vi "Initialize.vi"(8 "error in (no error)":errorcluster, 11 "VISA resource name":refnum<visa-resource-name>) -> (0 "error out":errorcluster, 3 "VISA resource name out":refnum<visa-resource-name>)   [LabVIEW 2023, in "JY-SPEX-TRIAX.lvlib"]
doc: "Establishes communication with the spectrometer; if the spectrometer hasn't yet been initialized, it does so. Generally, you need to call the Initialize VI only if the spectrometer has been powered off."
uses:
  JY-SPEX-TRIAX.lvlib
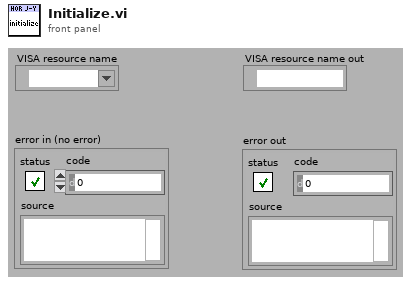
[diagram p1: front panel]
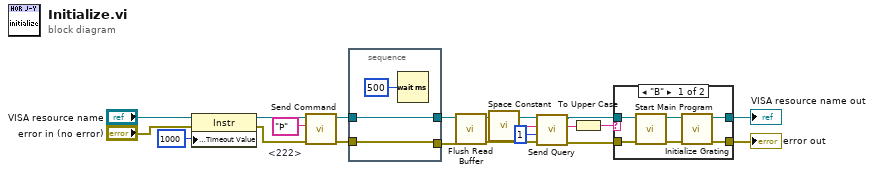
[diagram p0: block diagram]
diagram:
  w9 = "Þ"  # <222>
  n1 = property class="Instr"(reference="VISA resource name", error in="error in (no error)", "General Settings:Timeout Value"=u32 1000) -> (reference out=w14:refnum<visa-resource-name>, error out=w12:errorcluster)
  n2 = call "Send Command.vi"("error in (no error)"=w12, "write buffer"=w9, "VISA resource name"=w14) -> ("error out"=w11:errorcluster, "VISA resource name out"=w13:refnum<visa-resource-name>)  [unwired: 7 out]
  n3 = stacked-sequence {
    tunnel: w13 -> [w23]
    tunnel: [w23] -> w16
    tunnel: w11 -> [w21]
    tunnel: [w21] -> w10
    frame #0 {
      n4 = Wait (ms)(milliseconds to wait=u32 500) -> ()  [unwired: 1 out]
    }
  }
  n5 = call "Flush Read Buffer.vi"("error in (no error)"=w10, "VISA resource name"=w16) -> ("error out"=w4:errorcluster, "VISA resource name out"=w5:refnum<visa-resource-name>)  [unwired: 8 out]
  n6 = call <vilib>:"Space Constant.vi"() -> ("String"=w7:string)
  n7 = call "Send Query.vi"("error in (no error)"=w4, "byte count"=u32 1, "write buffer"=w7, "VISA resource name"=w5) -> ("error out"=w2:errorcluster, "read buffer"=w1:string, "VISA resource name out"=w3:refnum<visa-resource-name>)  [unwired: 5 out]
  n8 = To Upper Case(1:w1) -> (0:w19:string)
  n9 = case shown="\"B\"" w19 {
    tunnel: w3 -> [w29 w31]
    tunnel: w2 -> [w28 w30]
    tunnel: [w25 w31] -> w17
    tunnel: [w24 w30] -> w18
    frame "B" {
      n10 = call "Start Main Program.vi"("error in (no error)"=w28, "VISA resource name"=w29) -> ("error out"=w26:errorcluster, "VISA resource name out"=w27:refnum<visa-resource-name>)  [unwired: 8 out]
      n11 = call "Initialize Grating.vi"("error in (no error)"=w26, "VISA resource name"=w27) -> ("error out"=w24:errorcluster, "VISA resource name out"=w25:refnum<visa-resource-name>)  [unwired: 8 out]
    }
    frame "F", Default {
    }
  }
  "VISA resource name out" <- w17
  "error out" <- w18
